vi "Set DataType.vi"(8 "error in":errorcluster, 10 "Value":refnum<class "Value.lvclass">, 11 "DOMAIN in":refnum<class "DOMAIN.lvclass">) -> (0 "error out":errorcluster, 3 "DOMAIN out":refnum<class "DOMAIN.lvclass">)   [LabVIEW 2019, in "Electronic Datasheet.lvlib" / "DOMAIN.lvclass"]
uses:
  DOMAIN.lvclass
  Value/Value.lvclass
  Object Type/Object Type Base.lvclass
  Electronic Datasheet.lvlib
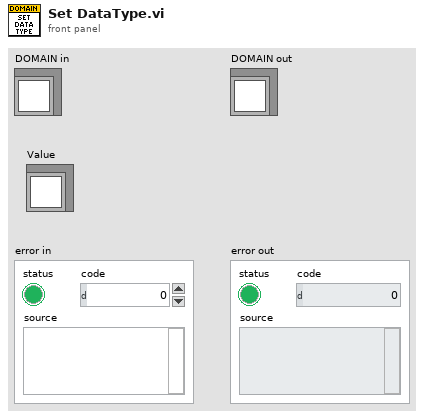
[diagram p1: front panel]
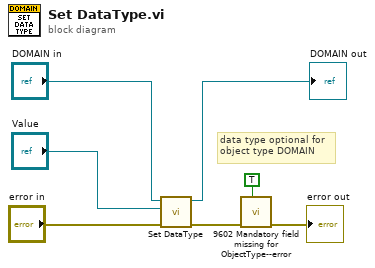
[diagram p0: block diagram]
diagram:
  # "data type optional for\nobject type DOMAIN"
  n1 = call-parent "Set DataType.vi"("error in"="error in", "Value"="Value", "Object Type in"="DOMAIN in") -> ("error out"=w6:errorcluster, "Object Type out"=→"DOMAIN out":refnum<class "DOMAIN.lvclass">)  [unwired: 7 in]
  n2 = call "9602 Mandatory field missing for ObjectType--error.vi"("Clear this Error?"=TRUE, "error in"=w6) -> ("error out"=→"error out":errorcluster)  [unwired: 9 in]
